vi "Open Waveform Sessions.vi"(8 "error in":errorcluster, 11 "Parameters":T4) -> (0 "error out":errorcluster, 2 "Injection.Results":T1 {"Measurements"."Shots"."Results"."Off-Stage Min Volt" format="%#.6g"; "Measurements"."Shots"."Results"."Off-Stage Avg Volt" format="%#.6g"; "Measurements"."Shots"."Results"."Off-Stage Max Volt" format="%#.6g"; "Measurements"."Shots"."Results"."Total Stage Time (us)" format="%#.6g"; "Measurements"."Shots"."Results"."Off-Stage Avg Current" format="%#.6g"; "Measurements"."Shots"."Results"."Total Voltage Pulses" format="%#.6g"; "Measurements"."Shots"."Results"."Off-Stage Min Current" format="%#.6g"; "Measurements"."Shots"."Results"."Off-Stage Max Current" format="%#.6g"}, 3 "Parameters":T4)   [LabVIEW 2019, in "Fuel Injector Analysis Addon Engine.lvlib"]
uses:
  Fuel Injector Analysis Addon Engine.lvlib
  Types/Async Parameters.ctl
  Addon Shared/Types/Shot.Parameters.ctl
  Addon Shared/Types/Stage.Parameters.ctl
  Addon Shared/Types/Stage.PullIn.Types.ctl
  Addon Shared/Types/Stage.Transition.Types.ctl
  Addon Shared/Types/Analysis.Channels.Select.ctl
  Addon Shared/Types/Injector info.ctl
  Types/Injector.State.ctl
  <vilib>/NI/NIVS Inline Async API/_Data Access Engine/Data Access Engine/Types/Write.DVR.ctl
  <vilib>/NI/NIVS Inline Async API/_Data Access Engine/Access Type Classes/Write/Write.lvclass
  <vilib>/NI/NIVS Inline Async API/_Data Access Engine/Data Access Engine/Types/Read.DVR.ctl
  <vilib>/NI/NIVS Inline Async API/_Data Access Engine/Access Type Classes/Read/Read.lvclass
  Addon Shared/Types/Compiled.Group.WaveformRefs.ctl
  <vilib>/NI VeriStand/Custom Device API/Waveform Data Reference.ctl
  <vilib>/NI VeriStand/Custom Device Waveform API/Single Waveform Write (DBL)/Single Waveform Write (DBL).lvclass
  Types/Injector Event Data Cluster.ctl
  Types/Shot Information Control.ctl
  Types/Stage.Measurements.ctl
  <vilib>/NI VeriStand/Custom Device Waveform API/Communication Properties.ctl
  Addon Shared/SubVIs/Constants.vi
  <vilib>/NI VeriStand/Custom Device Waveform API/Single Waveform Write (DBL)/NI VeriStand - Open Single Waveform Write Session (DBL).vi
  <vilib>/NI VeriStand/Custom Device Waveform API/NI_VS Custom Device Waveform API.lvlib
  Addon Shared/Fuel Injector Analysis Addon Shared.lvlib
  <vilib>/NI VeriStand/Custom Device API/Custom Device API.lvlib
  <vilib>/NI/NIVS Inline Async API/_Data Access Engine/Data Access Engine/Data Access Engine.lvclass
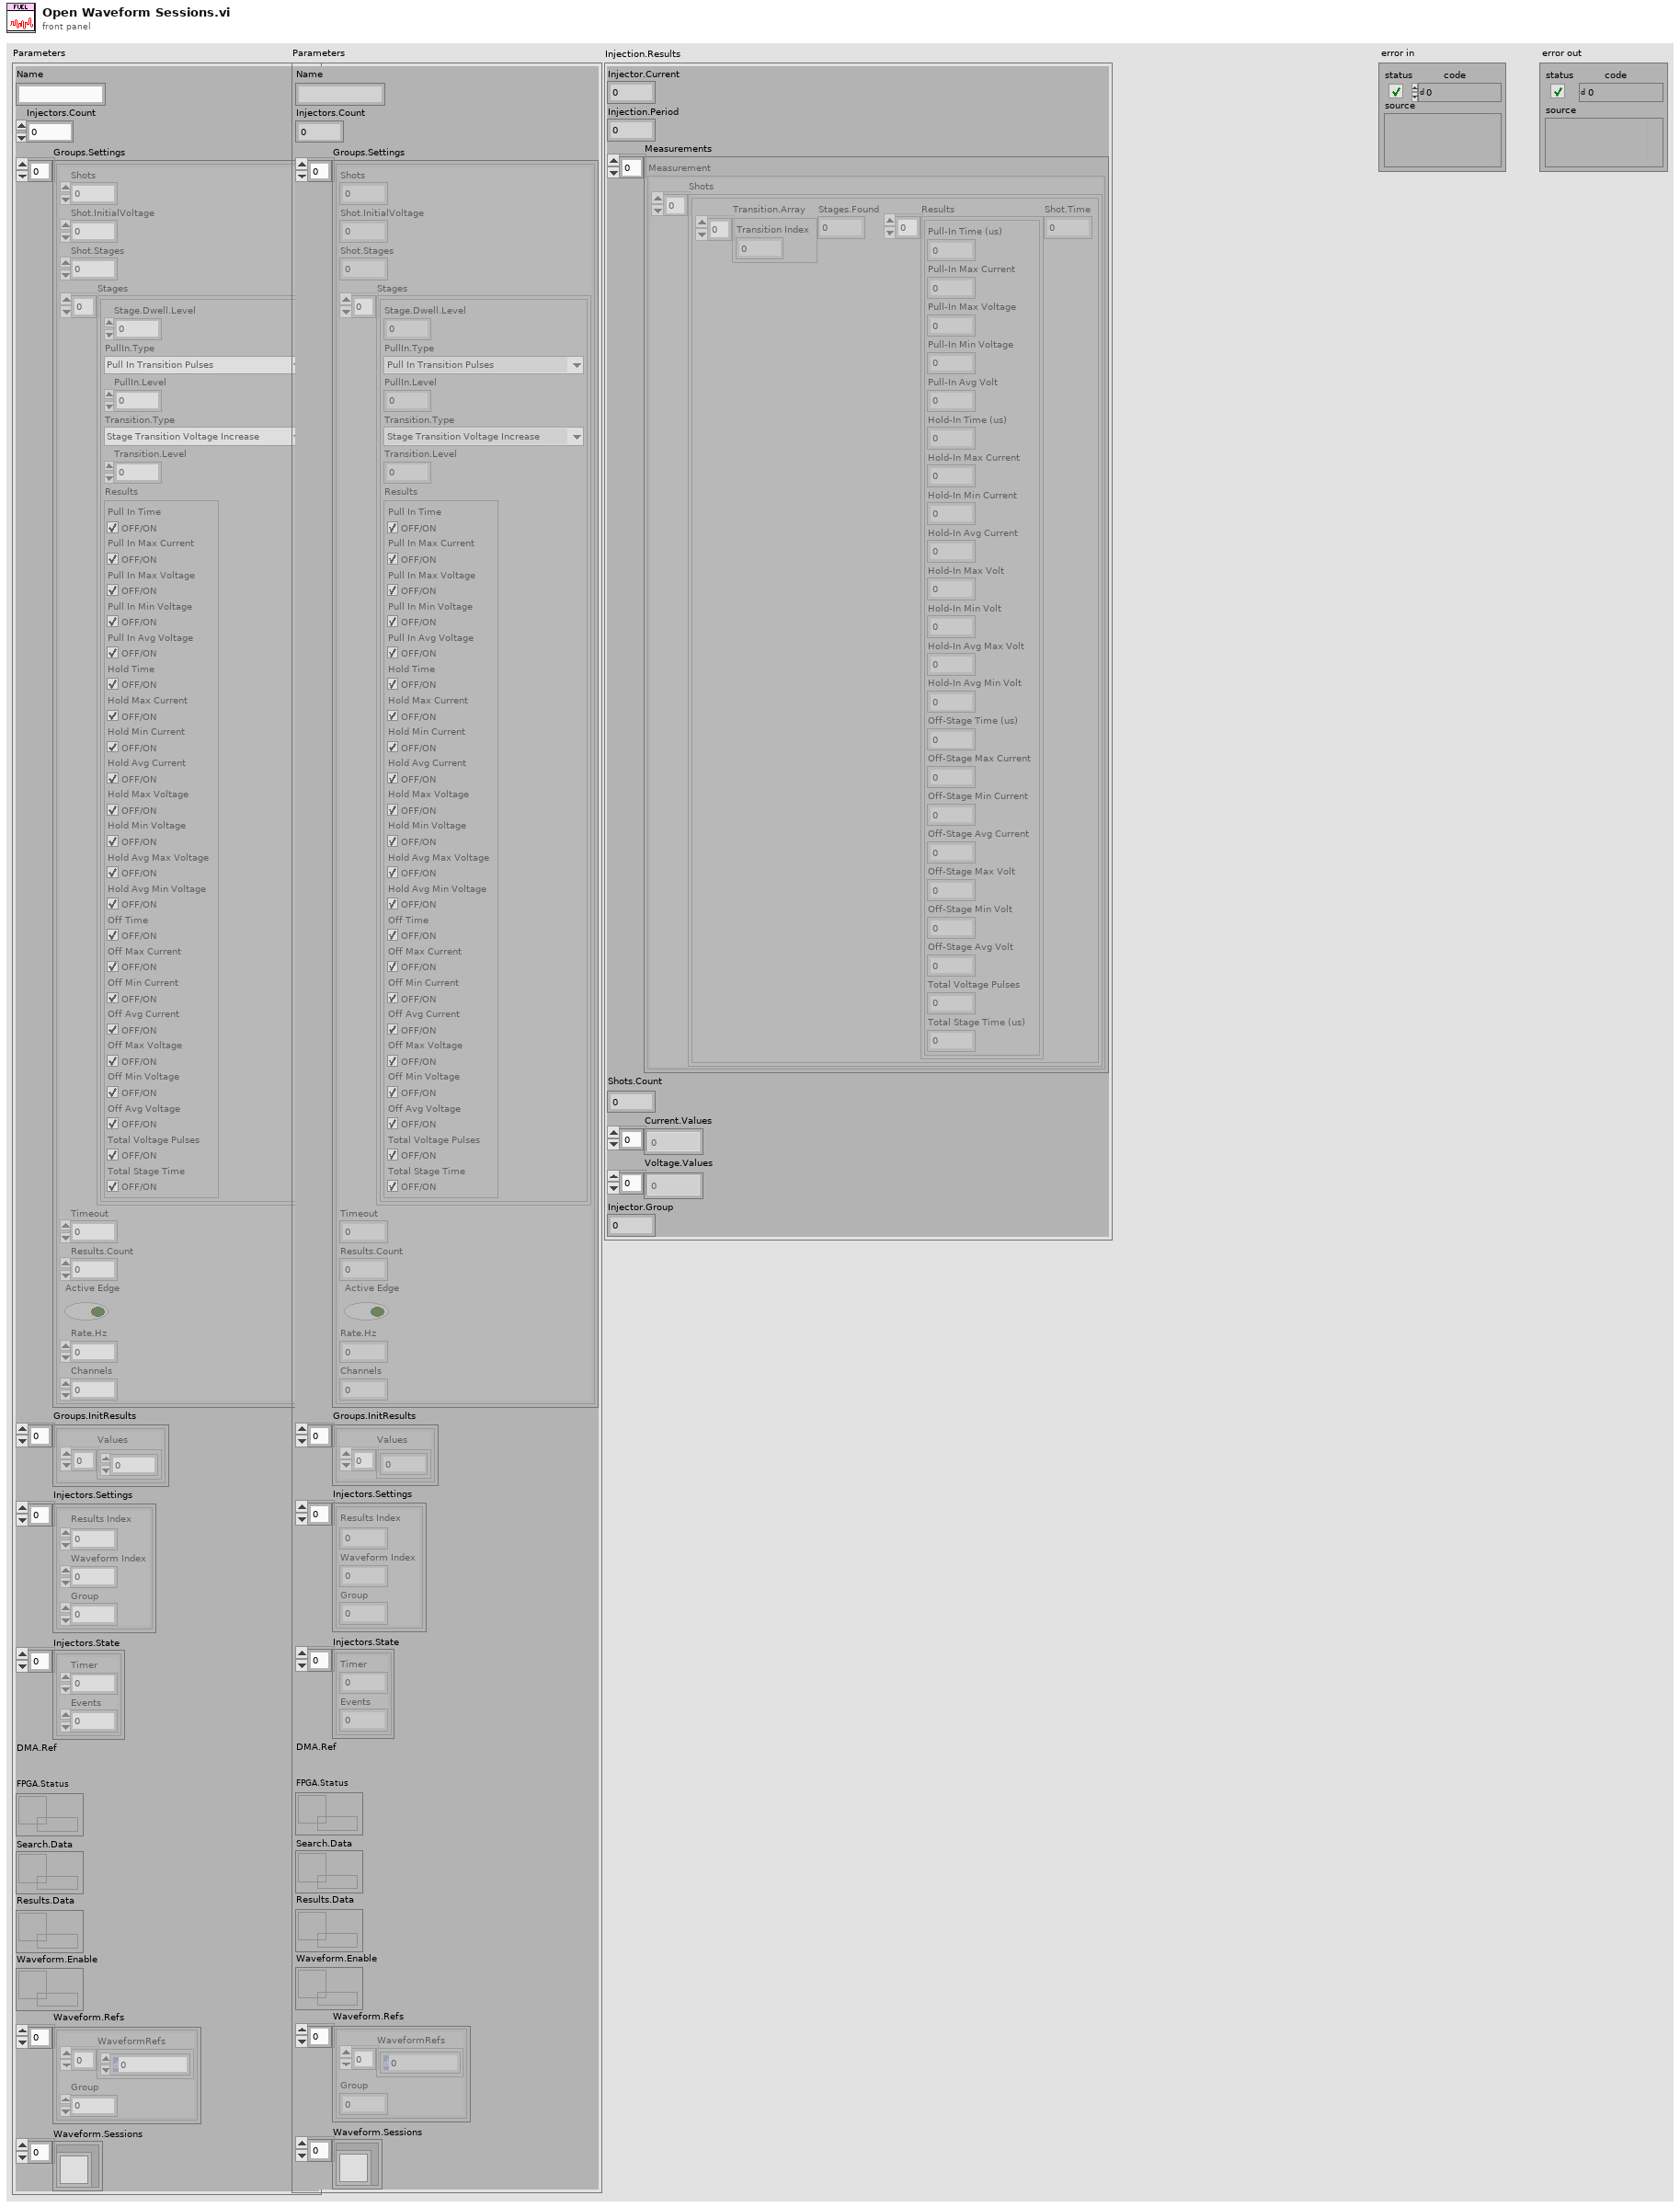
[diagram p1: front panel]
types:
  T1 = typedef "Fuel Injector Analysis Addon Engine.lvlib/Injector Event Data Cluster.ctl" = cluster{"Injector.Current":i16, "Injection.Period":dbl, "Measurements":cluster{"Shots":T2[]}[], "Shots.Count":i32, "Current.Values":dbl[], "Voltage.Values":dbl[], "Injector.Group":i16}
  T2 = typedef "Fuel Injector Analysis Addon Engine.lvlib/Shot Information Control.ctl" = cluster{"Transition.Array":i32[], "Stages.Found":u16, "Results":T3[], "Shot.Time":dbl}
  T3 = typedef "Fuel Injector Analysis Addon Engine.lvlib/Stage.Measurements.ctl" = cluster{"Pull-In Time (us)":dbl, "Pull-In Max Current":dbl, "Pull-In Max Voltage":dbl, "Pull-In Min Voltage":dbl, "Pull-In Avg Volt":dbl, "Hold-In Time (us)":dbl, "Hold-In Max Current":dbl, "Hold-In Min Current":dbl, "Hold-In Avg Current":dbl, "Hold-In Max Volt":dbl, "Hold-In Min Volt":dbl, "Hold-In Avg Max Volt":dbl, "Hold-In Avg Min Volt":dbl, "Off-Stage Time (us)":dbl, "Off-Stage Max Current":dbl, "Off-Stage Min Current":dbl, "Off-Stage Avg Current":dbl, "Off-Stage Max Volt":dbl, "Off-Stage Min Volt":dbl, "Off-Stage Avg Volt":dbl, "Total Voltage Pulses":dbl, "Total Stage Time (us)":dbl}
  T4 = typedef "Fuel Injector Analysis Addon Engine.lvlib/Async Parameters.ctl" = cluster{"Name":string, "Injectors.Count":u8, "Groups.Settings":T5[], "Groups.InitResults":cluster{"Values":dbl[]}[], "Injectors.Settings":T10[], "Injectors.State":T11[], "DMA.Ref":refnum<k20>, "FPGA.Status":T12, "Search.Data":T13, "Results.Data":T12, "Waveform.Enable":T13, "Waveform.Refs":T14[], "Waveform.Sessions":refnum<class "Single Waveform Write (DBL).lvclass">[]}
  T5 = typedef "Fuel Injector Analysis Addon Shared.lvlib/Shot.Parameters.ctl" = cluster{"Shots":u32, "Shot.InitialVoltage":dbl, "Shot.Stages":u32, "Stages":T6[], "Timeout":dbl, "Results.Count":i32, "Active Edge":bool, "Rate.Hz":u32, "Channels":u32}
  T6 = typedef "Fuel Injector Analysis Addon Shared.lvlib/Stage.Parameters.ctl" = cluster{"Stage.Dwell.Level":dbl, "PullIn.Type":T7, "PullIn.Level":dbl, "Transition.Type":T8, "Transition.Level":dbl, "Results":T9}
  T7 = typedef "Fuel Injector Analysis Addon Shared.lvlib/Stage.PullIn.Types.ctl" = enum8{"Pull In Transition Pulses", "Pull In Transition Current Drop"}
  T8 = typedef "Fuel Injector Analysis Addon Shared.lvlib/Stage.Transition.Types.ctl" = enum8{"Stage Transition Inactive Time", "Stage Transition Voltage Increase", "Stage Transition Current Decrease", "Stage Transition Active Time"}
  T9 = typedef "Fuel Injector Analysis Addon Shared.lvlib/Analysis.Channels.Select.ctl" = cluster{"Pull In Time":bool, "Pull In Max Current":bool, "Pull In Max Voltage":bool, "Pull In Min Voltage":bool, "Pull In Avg Voltage":bool, "Hold Time":bool, "Hold Max Current":bool, "Hold Min Current":bool, "Hold Avg Current":bool, "Hold Max Voltage":bool, "Hold Min Voltage":bool, "Hold Avg Max Voltage":bool, "Hold Avg Min Voltage":bool, "Off Time":bool, "Off Max Current":bool, "Off Min Current":bool, "Off Avg Current":bool, "Off Max Voltage":bool, "Off Min Voltage":bool, "Off Avg Voltage":bool, "Total Voltage Pulses":bool, "Total Stage Time":bool}
  T10 = typedef "Fuel Injector Analysis Addon Shared.lvlib/Injector info.ctl" = cluster{"Results Index":i32, "Waveform Index":i32, "Group":u16}
  T11 = typedef "Fuel Injector Analysis Addon Engine.lvlib/Injector.State.ctl" = cluster{"Timer":u32, "Events":u64}
  T12 = typedef "Data Access Engine.lvlib/Data Access Engine.lvclass/Write.DVR.ctl" = refnum<data-value>
  T13 = typedef "Data Access Engine.lvlib/Data Access Engine.lvclass/Read.DVR.ctl" = refnum<data-value>
  T14 = typedef "Fuel Injector Analysis Addon Shared.lvlib/Compiled.Group.WaveformRefs.ctl" = cluster{"WaveformRefs":T15[], "Group":i32}
  T15 = typedef "Custom Device API.lvlib/Waveform Data Reference.ctl" = i32
  T16 = typedef "NI_VS Custom Device Waveform API.lvlib/Communication Properties.ctl" = cluster{"WPL":cluster{"Custom Queue Size":i32, "Use Custom Queue Size?":bool}}
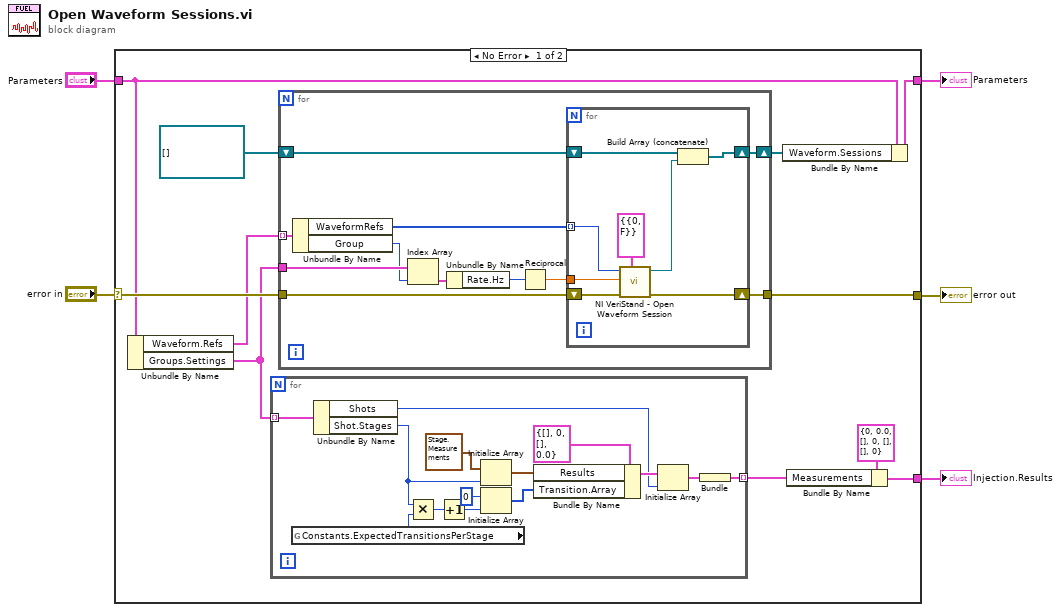
[diagram p0: block diagram]
diagram:
  n1 = case shown="No Error" "error in" {
    selector: "error in" -> [w16 w51]
    tunnel: "Parameters" -> [w13 w50]
    tunnel: [w15 w51] -> w4
    tunnel: [w12 w50] -> w2
    tunnel: [w10 _] -> w1
    frame No Error {
      n2 = Unbundle By Name(w13) -> ("Waveform.Refs"=w14:T14[], "Groups.Settings"=w8:T5[])
      n3 = for {
        tunnel: w8 -> [w21] mode=indexing
        tunnel: [w19] -> w9 mode=indexing
        n4 = global read "Constants.vi" "Constants.ExpectedTransitionsPerStage"() -> (w23:u32)
        n5 = Unbundle By Name(w21) -> ("Shots"=w17:u32, "Shot.Stages"=w18:u32)
        n6 = Multiply(x=w18, y=w23) -> (x*y=w26:u32)
        n7 = Increment(x=w26) -> (x+1=w22:u32)
        n8 = Initialize Array(T3 {"Pull-In Time (us)"=0.0, "Pull-In Max Current"=0.0, "Pull-In Max Voltage"=0.0, "Pull-In Min Voltage"=0.0, "Pull-In Avg Volt"=0.0, "Hold-In Time (us)"=0.0, "Hold-In Max Current"=0.0, "Hold-In Min Current"=0.0, "Hold-In Avg Current"=0.0, "Hold-In Max Volt"=0.0, "Hold-In Min Volt"=0.0, "Hold-In Avg Max Volt"=0.0, "Hold-In Avg Min Volt"=0.0, "Off-Stage Time (us)"=0.0, "Off-Stage Max Current"=0.0, "Off-Stage Min Current"=0.0, "Off-Stage Avg Current"=0.0, "Off-Stage Max Volt"=0.0, "Off-Stage Min Volt"=0.0, "Off-Stage Avg Volt"=0.0, "Total Voltage Pulses"=0.0, "Total Stage Time (us)"=0.0} ("Boost Stage Current Measurements"), w18) -> (w28:T3[])
        n9 = Initialize Array(0 ("Transition Index"), w22) -> (w24:i32[])
        n10 = Bundle By Name(cluster=T2 {"Transition.Array"=[], "Stages.Found"=0, "Results"=[], "Shot.Time"=0.0} ("Shot Info"), "Results"=w28, "Transition.Array"=w24) -> (w27:T2)
        n11 = Initialize Array(w27, w17) -> (w20:T2[])
        n12 = Bundle(w20) -> (w19:cluster{T2[]})  [unwired: 1 in]
      }
      n13 = for {
        tunnel: w16 -> [w41]
        tunnel: [w40] -> w15
        tunnel: w14 -> [w39] mode=indexing
        tunnel: w8 -> [w37]
        shift-right: [w31] -> w6
        shift-left: refnum<class "Single Waveform Write (DBL).lvclass">[] [] -> [w32]
        n14 = Unbundle By Name(w39) -> ("WaveformRefs"=w33:T15[], "Group"=w36:i32)
        n15 = Index Array(array=w37, index=w36) -> (element=w35:T5)
        n16 = Unbundle By Name(w35) -> ("Rate.Hz"=w34:u32)
        n17 = Reciprocal(x=w34) -> (1/x=w38:dbl)
        n18 = for {
          tunnel: w38 -> [w46]
          shift-right: [w48] -> w40
          shift-left: w41 -> [w49]
          tunnel: w33 -> [w45] mode=indexing
          shift-right: [w42] -> w31
          shift-left: w32 -> [w44]
          n19 = call-poly <vilib>:"NI VeriStand - Open Waveform Session.vi"("Communication Properties"=T16 {"WPL"={"Custom Queue Size"=0, "Use Custom Queue Size?"=FALSE}}, "error in (no error)"=w49, "dt"=w46, "DBL Waveform Data Reference"=w45) -> ("error out"=w48:errorcluster, "Single Waveform Write Session (DBL)"=w43:refnum<class "Single Waveform Write (DBL).lvclass">)  [unwired: 6 in]
          n20 = Build Array (concatenate)(w44, w43) -> (w42:refnum<class "Single Waveform Write (DBL).lvclass">[])
        }
      }
      n21 = Bundle By Name(cluster=w13, "Waveform.Sessions"=w6) -> (w12:T4)
      n22 = Bundle By Name(cluster=T1 {"Injector.Current"=0, "Injection.Period"=0.0, "Measurements"=[], "Shots.Count"=0, "Current.Values"=[], "Voltage.Values"=[], "Injector.Group"=0} ("Injection Event Data Cluster in"), "Measurements"=w9) -> (w10:T1)
    }
    frame Error {
    }
  }
  "error out" <- w4
  "Parameters" <- w2
  "Injection.Results" <- w1
